vi "Esercitazione 5 - Array e Matrici.vi"() -> ()   [LabVIEW 2018]
panel:
  out "output array":dbl[][](array[numeric])
  in  "new element/subarray":dbl[](array[numeric])
  in  "index (row)":i32
  in  "Array":dbl[][](array[numeric])
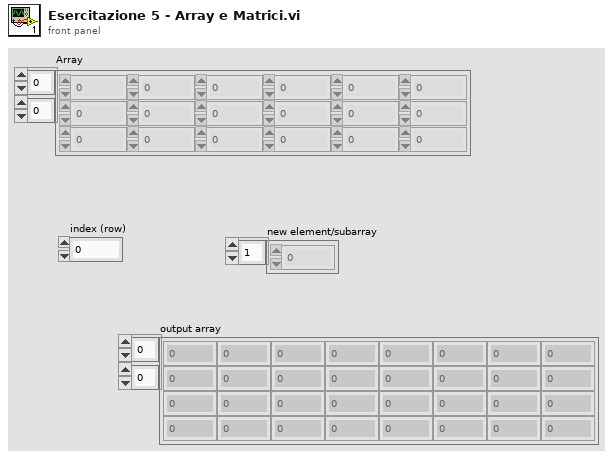
[diagram p1: front panel]
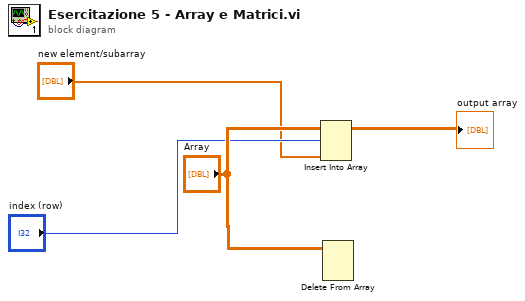
[diagram p0: block diagram]
diagram:
  n1 = Insert Into Array "Insert Into Array"(array="Array", index (row)="index (row)", new element="new element/subarray") -> (→"output array":dbl[][])  [unwired: 1 in]
  n2 = Delete From Array "Delete From Array"(array="Array") -> ()  [unwired: 3 in, 2 out]
